vi "integral_power.vi"(0 "Temp":dbl, 7 "Control Parameters":T1={"Setpoint"=50.0, "Control bandwidth"=4.0, "Settle bandwidth"=1.0, "Integral time"=30.0, "Int\non"=TRUE, "Derivative time"=0.5, "Der\non"=TRUE, "Settle time"=60.0} {"Settle time" format="%.2f"; "Derivative time" format="%.2f"; "Integral time" format="%.2f"; "Settle bandwidth" format="%.2f"; "Control bandwidth" format="%.2f"; "Setpoint" format="%.2f"}, 11 "Reset PID":bool, 13 "Elapsed Time":dbl) -> (4 "Normalized Power":dbl)   [LabVIEW 2016]
uses:
  typedefs/control parameters.ctl
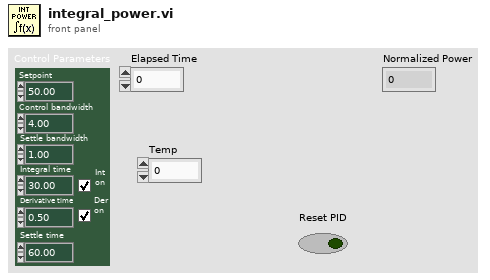
[diagram p1: front panel]
types:
  T1 = typedef "control parameters.ctl" = cluster{"Setpoint":dbl, "Control bandwidth":dbl, "Settle bandwidth":dbl, "Integral time":dbl, "Int\non":bool, "Derivative time":dbl, "Der\non":bool, "Settle time":dbl}
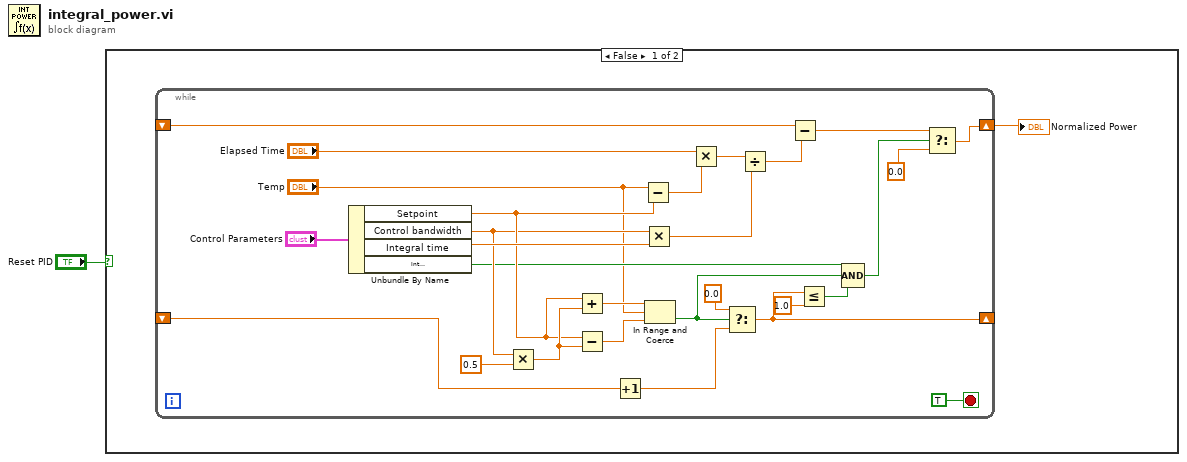
[diagram p0: block diagram]
diagram:
  n1 = case shown="False" "Reset PID" {
    frame False {
      n2 = while {
        shift-right: [w7] -> w2
        shift-left: _ -> [w26]
        shift-right: [w4] -> _
        shift-left: _ -> [w13]
        stop <- TRUE stop-if-true
        n3 = Unbundle By Name("Control Parameters") -> ("Setpoint"=w21:dbl, "Control bandwidth"=w20:dbl, "Integral time"=w28:dbl, "Int\non"=w16:bool)
        n4 = Multiply(x=w20, y=0.5) -> (x*y=w22:dbl)
        n5 = Add(x=w21, y=w22) -> (x+y=w19:dbl)
        n6 = Subtract(x=w21, y=w22) -> (x-y=w18:dbl)
        n7 = Increment(x=w13) -> (x+1=w12:dbl)
        n8 = Subtract(x="Temp", y=w21) -> (x-y=w30:dbl)
        n9 = Multiply(x=w20, y=w28) -> (x*y=w27:dbl)
        n10 = In Range and Coerce(upper limit=w19, x="Temp", lower limit=w18) -> (In Range?=w15:bool)  [unwired: 1 out]
        n11 = Multiply(x="Elapsed Time", y=w30) -> (x*y=w29:dbl)
        n12 = Select(t=0.0, s=w15, f=w12) -> (s? t:f=w4:dbl)
        n13 = Divide(x=w29, y=w27) -> (x/y=w25:dbl)
        n14 = Subtract(x=w26, y=w25) -> (x-y=w8:dbl)
        n15 = Less Or Equal?(x=w4, y=1.0) -> (x <= y?=w5:bool)
        n16 = Compound Arithmetic op=AND(w16, w15, w5) -> (w9:bool)
        n17 = Select(t=w8, s=w9, f=0.0) -> (s? t:f=w7:dbl)
      }
      "Normalized Power" <- w2
    }
    frame True {
    }
  }
